vi "Experiment-2-4-2.vi"() -> ()   [LabVIEW 2014]
panel:
  out "Resistor Value":dbl
  in  "3d Band":T1(ring)
  in  "2nd Band":T1(ring)
  in  "1st Band":T1(ring)
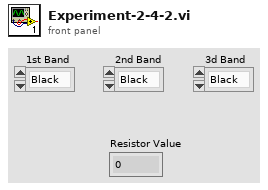
[diagram p1: front panel]
types:
  T1 = enum16{"Black", "Brown", "Red", "Orange", "Yellow", "Green", "Blue", "Purple", "Gray", "White"}
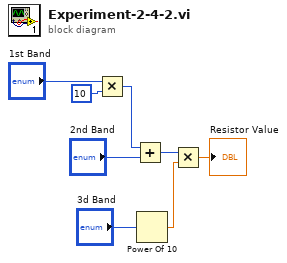
[diagram p0: block diagram]
diagram:
  n1 = Multiply(x="1st Band", y=10) -> (x*y=w6:i32)
  n2 = Add(x=w6, y="2nd Band") -> (x+y=w3:i32)
  n3 = Power Of 10(x="3d Band") -> (10^x=w2:dbl)
  n4 = Multiply(x=w3, y=w2) -> (x*y=→"Resistor Value":dbl)
